vi "RX.vi"(1 "aDATA":u8[](array[numeric])) -> (0 "Boolean array":bool[](array[boolean]))   [LabVIEW 2016]
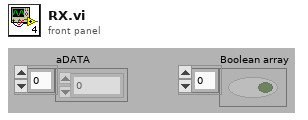
[diagram p1: front panel]
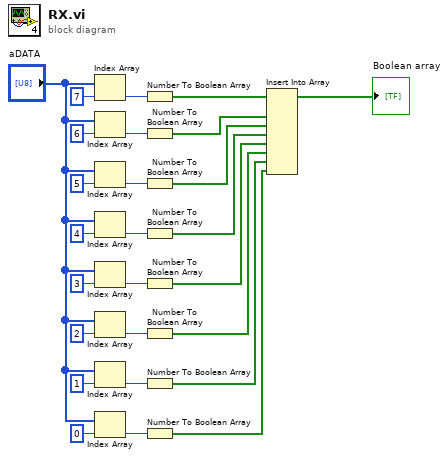
[diagram p0: block diagram]
diagram:
  n1 = Index Array(array="aDATA", index=7) -> (element=w10:u8)
  n2 = Index Array(array="aDATA", index=6) -> (element=w12:u8)
  n3 = Index Array(array="aDATA", index=5) -> (element=w13:u8)
  n4 = Index Array(array="aDATA", index=4) -> (element=w11:u8)
  n5 = Index Array(array="aDATA", index=3) -> (element=w14:u8)
  n6 = Index Array(array="aDATA", index=2) -> (element=w15:u8)
  n7 = Index Array(array="aDATA", index=1) -> (element=w16:u8)
  n8 = Index Array(array="aDATA", index=0) -> (element=w17:u8)
  n9 = Number To Boolean Array(number=w10) -> (Boolean array=w18:bool[])
  n10 = Number To Boolean Array(number=w12) -> (Boolean array=w19:bool[])
  n11 = Number To Boolean Array(number=w13) -> (Boolean array=w20:bool[])
  n12 = Number To Boolean Array(number=w11) -> (Boolean array=w21:bool[])
  n13 = Number To Boolean Array(number=w14) -> (Boolean array=w22:bool[])
  n14 = Number To Boolean Array(number=w15) -> (Boolean array=w23:bool[])
  n15 = Number To Boolean Array(number=w16) -> (Boolean array=w24:bool[])
  n16 = Number To Boolean Array(number=w17) -> (Boolean array=w25:bool[])
  n17 = Insert Into Array(array=w18, new element #1=w19, new element #2=w20, new element #3=w21, new element #4=w22, new element #5=w23, new element #6=w24, new element #7=w25) -> (→"Boolean array":bool[])  [unwired: 1 in]
